vi "氨氮加标回收 (子VI).vi"(11 "是否启动对话框":bool) -> ()   [LabVIEW 2016, in "质控单元.lvlib"]
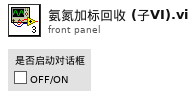
[diagram p1: front panel]
types:
  T1 = enum32{"Bad", "Idle", "Run top level", "Running"}
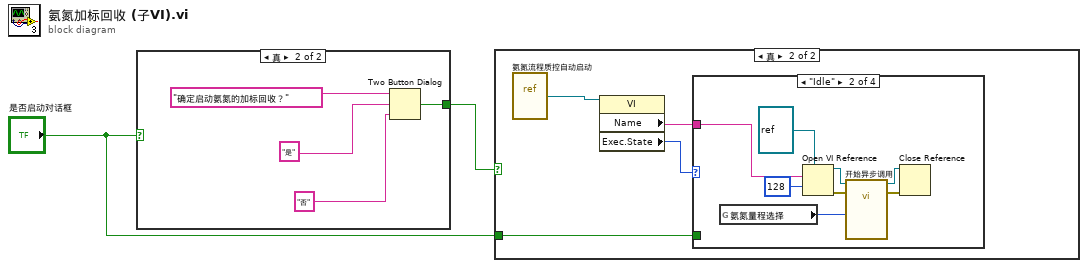
[diagram p0: block diagram]
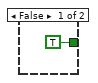
[diagram p2: hidden frame]
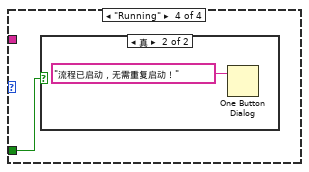
[diagram p6: hidden frame]
diagram:
  n1 = case shown="真" "是否启动对话框" {
    tunnel: [TRUE ("T button?") w7] -> w2
    frame False {
    }
    frame True {
      n2 = Two Button Dialog(message="确定启动氨氮的加标回收？" ("消息"), 1:"否" ("F按钮名称（“取消”）"), 2:"是" ("T按钮名称（“确定”）")) -> (T button?=w7:bool)
    }
  }
  n3 = case shown="真" w2 {
    tunnel: "是否启动对话框" -> [_ w8]
    frame False {
    }
    frame True {
      n4 = vi-ref "氨氮流程质控自动启动.vi"() -> (w11:refnum<vi>)
      n5 = property class="VI"(reference=w11) -> ("Name"=w9:string, "Exec.State"=w10:T1)  [unwired: 1 in, 2 out]
      n6 = case shown="\"Idle\"" w10 {
        tunnel: w9 -> [_ w15 _ _]
        tunnel: w8 -> [_ _ _ w20]
        frame "Bad", Default {
        }
        frame "Idle" {
          n7 = global read "断电保存全局.vi" "氨氮量程选择"() -> (w12:enum32{"H", "L", "AUTO"})
          n8 = Open VI Reference(type specifier VI Refnum (for type only)=refnum<vi> refnum ("类型说明符VI引用句柄（仅用于类型）"), vi path=w15, options=128 ("选项")) -> (vi reference=w19:refnum<vi>, error out=w14:errorcluster)  [unwired: 3 in]
          n9 = call-by-ref "开始异步调用"(reference=w19, error in=w14, "氨氮量程切换"=w12) -> (reference out=w18:refnum<vi>, error out=w13:errorcluster)  [unwired: 11 in]
          n10 = Close Reference(reference=w18, error in (no error)=w13) -> ()  [unwired: 1 out]
        }
        frame "Run top level" {
        }
        frame "Running" {
          n11 = case shown="真" w20 {
            frame False {
            }
            frame True {
              n12 = One Button Dialog(message="流程已启动，无需重复启动！" ("消息")) -> ()  [unwired: 1 in, 1 out]
            }
          }
        }
      }
    }
  }
